vi "OC2 Read Control.vi"(3 "error in (no error)":errorcluster, 4 "control type report in":T1 {"Power up state" items=["Off", "On", "Last"]; "Dead Band" format="%.2f"; "Derivative TC" format="%.1f"; "Derivative" format="%.2f"; "Integral" format="%.1f"; "Proportional Gain" format="%.1f"; "Control Type" items=["Off", "On/Off", "P", "PI", "PID"]}, 5 "enable":bool, 6 "VISA resource name":refnum<visa-resource-name>) -> (0 "error out":errorcluster, 1 "control type report out":T1 {"Power up state" items=["Off", "On", "Last"]; "Dead Band" format="%.2f"; "Derivative TC" format="%.1f"; "Derivative" format="%.2f"; "Integral" format="%.1f"; "Proportional Gain" format="%.1f"; "Control Type" items=["Off", "On/Off", "P", "PI", "PID"]}, 2 "dup VISA resource name":refnum<visa-resource-name>)   [LabVIEW 2009]
doc: "TCM Read Control.vi\n\nVI that reads the control information, accepts a cluster that contains the following variables:\nControl Type - off, PID etc\nProportional gain - control proportional gain (P term)\nIntergral - control integral (i term)\nDerivative - control derivative (D term)\nDerivative TC\nDead Band\nPower up state - off the control is not on when tcm starts, on control is on with tcm power up\n\nCOPYRIGHT ELECTRON DYNAMICS LTD"
panel:
  out "remaining string":string
  in  "Command":string
  out "Rx string":string
  # "Read Control data"
  # "V1.02"
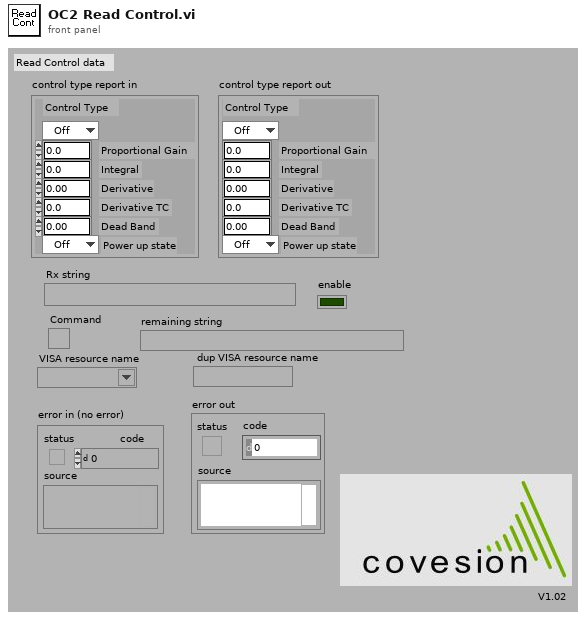
[diagram p1: front panel]
types:
  T1 = cluster{"Control Type":u16, "Proportional Gain":dbl, "Integral":dbl, "Derivative":dbl, "Derivative TC":dbl, "Dead Band":dbl, "Power up state ":u16}
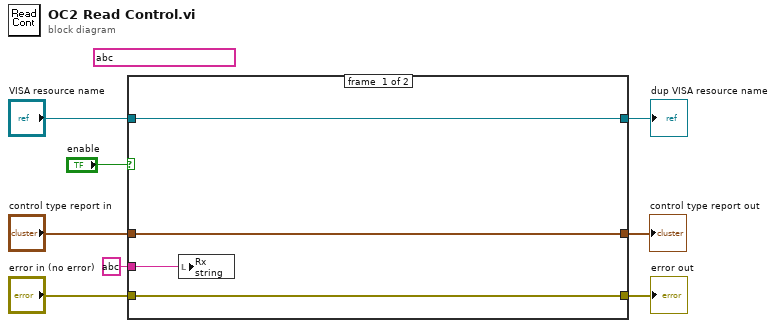
[diagram p0: block diagram]
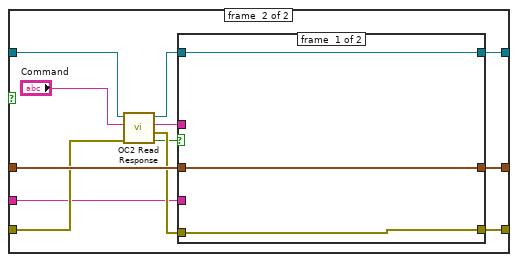
[diagram p2: hidden frame]
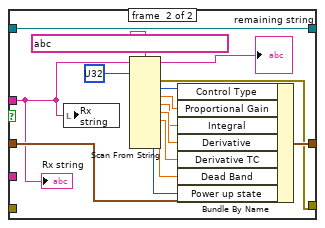
[diagram p3: hidden frame]
diagram:
  (unwired) string ? ("format string")
  n1 = case shown="True" "enable" {
    tunnel: "error in (no error)" -> [w11 w21]
    tunnel: "VISA resource name" -> [w12 w20]
    tunnel: [w11 w19] -> w6
    tunnel: [w12 w17] -> w5
    tunnel: [w10 w16] -> w4
    tunnel: "control type report in" -> [w10 w23]
    tunnel: string ? ("Rx string") -> [w9 w15]
    frame #0 {
      n2 = local write "Rx string"(w9) -> ()
    }
    frame #1 {
      n3 = call "OC2 Read Response.vi"("error in (no error)"=w21, "Command"="Command", "VISA resource name"=w20) -> ("RX packet ok"=w13:bool, "error out"=w22:errorcluster, "output string"=w14:string, "dup VISA resource name"=w18:refnum<visa-resource-name>)  [unwired: 1 in]
      n4 = case shown="True" w13 {
        tunnel: w14 -> [_ w28]
        tunnel: w23 -> [w25 w41]
        tunnel: w22 -> [w27 _]
        tunnel: [w27 w32] -> w19
        tunnel: w18 -> [w26 w35]
        tunnel: [w26 w35] -> w17
        tunnel: [w25 w33] -> w16
        tunnel: w15 -> [_ _]
        frame #0 {
        }
        frame #1 {
          n5 = local write "Rx string"(w28) -> ()
          n6 = Scan From String(format string=string ?, input string=w28, initial scan location=u32 ?) -> (remaining string=→"remaining string":string, error out=w32:errorcluster, output 1=w30:i32, output 2=w40:dbl, output 3=w34:dbl, output 4=w39:dbl, output 5=w38:dbl, output 6=w37:dbl, output 7=w36:i32)  [unwired: 10 in, 1 out]
          n7 = Bundle By Name(cluster=w41, "Control Type"=w30, "Proportional Gain"=w40, "Integral"=w34, "Derivative"=w39, "Derivative TC"=w38, "Dead Band"=w37, "Power up state"=w36) -> (w33:T1)
          "Rx string" <- w28
        }
      }
    }
  }
  "error out" <- w6
  "dup VISA resource name" <- w5
  "control type report out" <- w4
